vi "snap image.vi"() -> ()   [LabVIEW 2018]
uses:
  <vilib>/userdefined/High Color/IMAQdx.ctl
  <vilib>/vision/driver/NI_Vision_Acquisition_Software.lvlib
panel:
  in  "Session In":T1
  out "Image":T2(plugin-control)
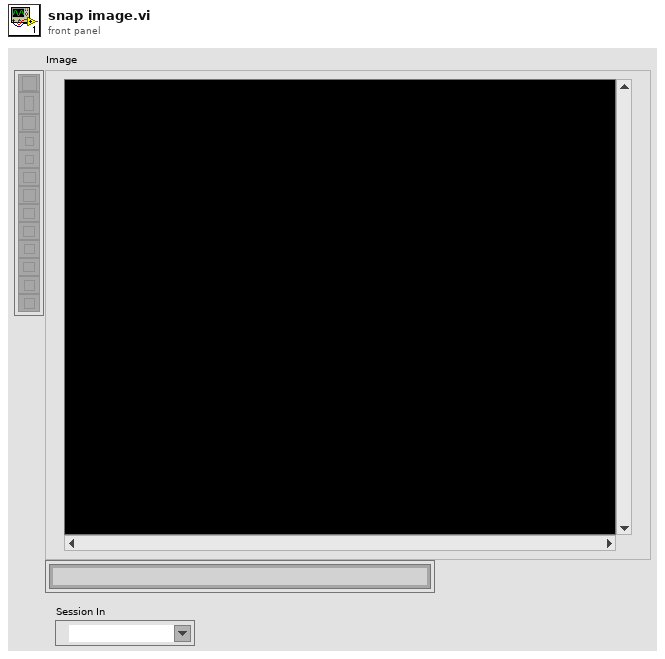
[diagram p1: front panel]
types:
  T1 = typedef "IMAQdx.ctl" = refnum<k21>
  T2 = typedef "IMAQ Image.ctl" = refnum<image>
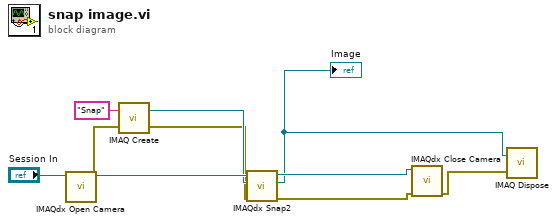
[diagram p0: block diagram]
diagram:
  n1 = call <vilib>:"IMAQdx Open Camera.vi"("Session In"="Session In") -> ("error out"=w4:errorcluster, "Session Out"=w10:T1)  [unwired: 9 in]
  n2 = call "IMAQ Create"("Image Name"="Snap", "error in (no error)"=w4) -> ("New Image"=w6:T2, "error out"=w3:errorcluster)  [unwired: 3 in]
  n3 = call <vilib>:"IMAQdx Snap2.vi"("error in"=w3, "Image In"=w6, "Session In"=w10) -> ("error out"=w8:errorcluster, "Image Out"=w2:T2, "Session Out"=w9:T1)  [unwired: 6 in]
  "Image" <- w2
  n4 = call <vilib>:"IMAQdx Close Camera.vi"("error in"=w8, "Session In"=w9) -> ("error out"=w1:errorcluster)  [unwired: 9 in]
  n5 = call "IMAQ Dispose"("Image"=w2, "error in (no error)"=w1) -> ()  [unwired: 4 in, 1 out]
